vi "getPublicEvents.vi"(8 "error in (no error)":errorcluster, 11 "TextTestRunner in":refnum<class "TestRunner.lvclass">) -> (0 "error out":errorcluster, 2 "publicEvents":T1, 3 "TextTestRunner out":refnum<class "TestRunner.lvclass">)   [LabVIEW 2011, in "TestRunner.lvclass"]
uses:
  TestRunner.lvclass
  PublicEvents--Cluster.ctl
  TestResult/resultStatusChanged--Cluster.ctl
  TestResult/resultStatus--enum.ctl
  TestResult/testStarted--Cluster.ctl
  TestRunner.lvclass/TestRunner.ctl
  TestResult/TestResult.lvclass
panel:
  # "JKI VI Tester for LabVIEW\nhttp://jkisoft.com/vi-tester\nCopyright (C) 2007-2009, JKI <info@jkisoft.com>\nALL RIGHTS RESERVED"
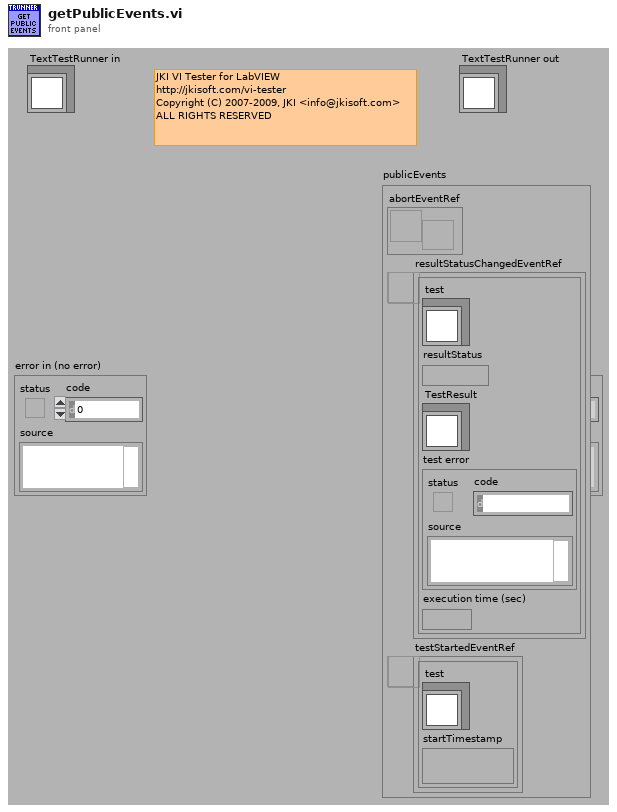
[diagram p1: front panel]
types:
  T1 = typedef "TestRunner.lvclass/PublicEvents--Cluster.ctl" = cluster{"abortEventRef":refnum<user-event>, "resultStatusChangedEventRef":refnum<user-event>, "testStartedEventRef":refnum<user-event>}
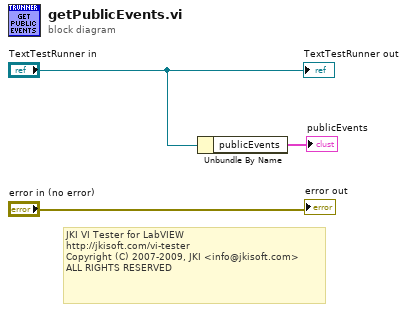
[diagram p0: block diagram]
diagram:
  # "JKI VI Tester for LabVIEW\nhttp://jkisoft.com/vi-tester\nCopyright (C) 2007-2009, JKI <info@jkisoft.com>\nALL RIGHTS RESERVED"
  n1 = Unbundle By Name("TextTestRunner in") -> ("publicEvents"=→"publicEvents":T1)
  "error out" <- "error in (no error)"
  "TextTestRunner out" <- "TextTestRunner in"
